vi "Drop.vi"(11 "element in":T1) -> ()   [LabVIEW 2019, in "MessengerM.lvlib" / "SubChannelCPU.lvclass"]
uses:
  SubChannelCPU.lvclass
  <vilib>/ChannelSupport/Channel Message/Channel Message.lvclass
  Element.ctl
  MessengerM.lvlib
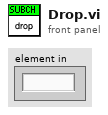
[diagram p1: front panel]
types:
  T1 = typedef "MessengerM.lvlib/Element.ctl" = string
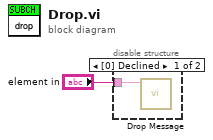
[diagram p0: block diagram]
diagram:
  n1 = disable-structure shown="[0] Declined" {
    disable-tunnel: "element in" -> [w2 _]
    frame Disabled {
      n2 = call-dynamic "Drop Message.vi"("Channel Message in"=w2) -> ()  [unwired: 10 in, 1 out]
    }
    frame Enabled {
    }
  }
